vi "AutoEject.vi"(8 "error in (no error)":errorcluster, 9 "Time":dbl, 10 "Left Flywheel DevRef":T1={"DeviceStatus"={"status"=FALSE, "code"=0, "source"=""}, "Type"=enum."PWM", "PWM"={"PWM Channel"=enum."Invalid", "DeadBand"={"Name"="", "maxPositivePwm"=0, "minPositivePwm"=0, "centerPwm"=0, "maxNegativePwm"=0, "minNegativePwm"=0, "angularRange"=0}}, "CAN"={"Device Number"=0, "SetOutput VI Ref"=variant, "GetOutput VI Ref"=variant, "Enable VI Ref"=variant, "Disable VI Ref"=variant, "Data"=variant}, "Invert"=FALSE, "DIO PWM"={"PWM \"Enable\" Channel"=enum."Invalid", "DIOChannel"=enum."Invalid", "PWM Rate"=0.0}}, 11 "Right Flywheel DevRef":T1={"DeviceStatus"={"status"=FALSE, "code"=0, "source"=""}, "Type"=enum."PWM", "PWM"={"PWM Channel"=enum."Invalid", "DeadBand"={"Name"="", "maxPositivePwm"=0, "minPositivePwm"=0, "centerPwm"=0, "maxNegativePwm"=0, "minNegativePwm"=0, "angularRange"=0}}, "CAN"={"Device Number"=0, "SetOutput VI Ref"=variant, "GetOutput VI Ref"=variant, "Enable VI Ref"=variant, "Disable VI Ref"=variant, "Data"=variant}, "Invert"=FALSE, "DIO PWM"={"PWM \"Enable\" Channel"=enum."Invalid", "DIOChannel"=enum."Invalid", "PWM Rate"=0.0}}) -> (0 "error out":errorcluster)   [LabVIEW 2017]
uses:
  <vilib>/Rock Robotics/WPI/MotorControl/WPI_MotorControlDeviceRef.ctl
  <vilib>/Rock Robotics/WPI/MotorControl/WPI_MotorControlType.ctl
  <vilib>/Rock Robotics/SystemInterfaces/DIO/FPGA_DIOPWMChannel.ctl
  <vilib>/Rock Robotics/WPI/PWM/WPI_PWMDeadband.ctl
  <vilib>/Rock Robotics/SystemInterfaces/DIO/FPGA_DIOChannel.ctl
  <vilib>/Rock Robotics/WPI/ThirdParty/Phoenix-LabVIEW/Motor Controller/Controls/CTRE_Phoenix_MotorControl_ControlMode.ctl
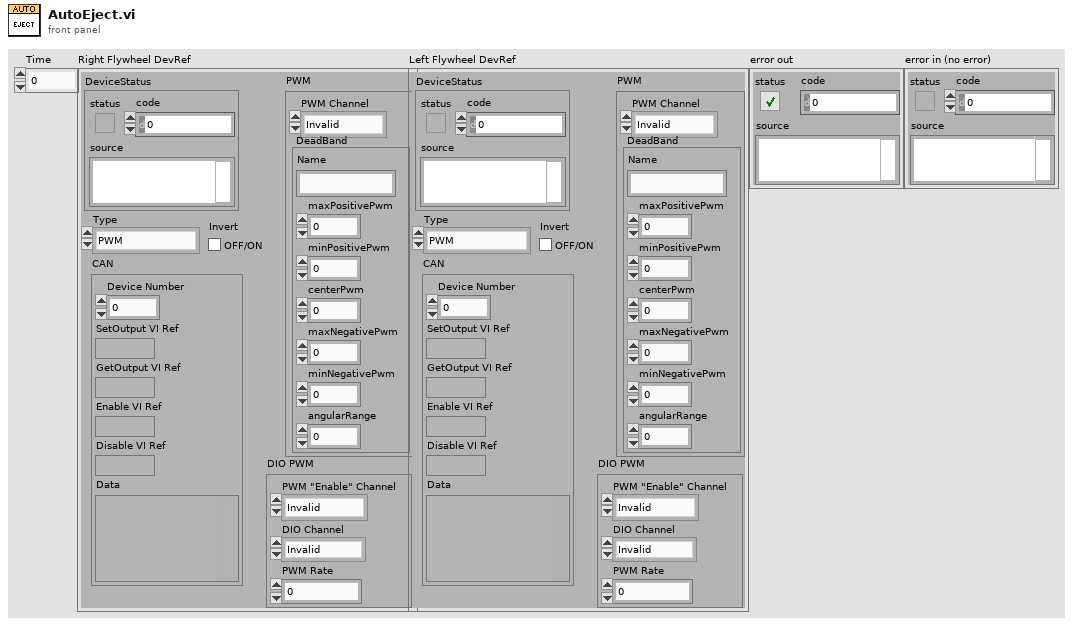
[diagram p1: front panel]
types:
  T1 = typedef "WPI_MotorControlDeviceRef.ctl" = cluster{"DeviceStatus":errorcluster, "Type":T2, "PWM":cluster{"PWM Channel":T3, "DeadBand":T4}, "CAN":cluster{"Device Number":u8, "SetOutput VI Ref":variant, "GetOutput VI Ref":variant, "Enable VI Ref":variant, "Disable VI Ref":variant, "Data":variant}, "Invert":bool, "DIO PWM":cluster{"PWM \"Enable\" Channel":T3, "DIOChannel":T5, "PWM Rate":dbl}}
  T2 = typedef "WPI_MotorControlType.ctl" = enum16{"PWM", "CAN", "DIO PWM"}
  T3 = typedef "FPGA_DIOPWMChannel.ctl" = enum8{"PWM 0", "PWM 1", "PWM 2", "PWM 3", "PWM 4", "PWM 5", "PWM 6", "PWM 7", "PWM 8", "PWM 9", "PWM MXP 0", "PWM MXP 1", "PWM MXP 2", "PWM MXP 3", "PWM MXP 4", "PWM MXP 5", "PWM MXP 6", "PWM MXP 7", "PWM MXP 8", "PWM MXP 9", "Invalid"}
  T4 = typedef "WPI_PWMDeadband.ctl" = cluster{"Name":string, "maxPositivePwm":i32, "minPositivePwm":i32, "centerPwm":i32, "maxNegativePwm":i32, "minNegativePwm":i32, "angularRange":u16}
  T5 = typedef "FPGA_DIOChannel.ctl" = enum8{"DIO 0", "DIO 1", "DIO 2", "DIO 3", "DIO 4", "DIO 5", "DIO 6", "DIO 7", "DIO 8", "DIO 9", "DIO MXP 0", "DIO MXP 1", "DIO MXP 2", "DIO MXP 3", "DIO MXP 4", "DIO MXP 5", "DIO MXP 6", "DIO MXP 7", "DIO MXP 8", "DIO MXP 9", "DIO MXP 10", "DIO MXP 11", "DIO MXP 12", "DIO MXP 13", "DIO MXP 14", "DIO MXP 15", "SPI Port CS1", "SPI Port CS2", "SPI Port CS3", "SPI Port MISO", "SPI Port MOSI", "Invalid"}
  T6 = typedef "CTRE_Phoenix_MotorControl_ControlMode.ctl" = u16
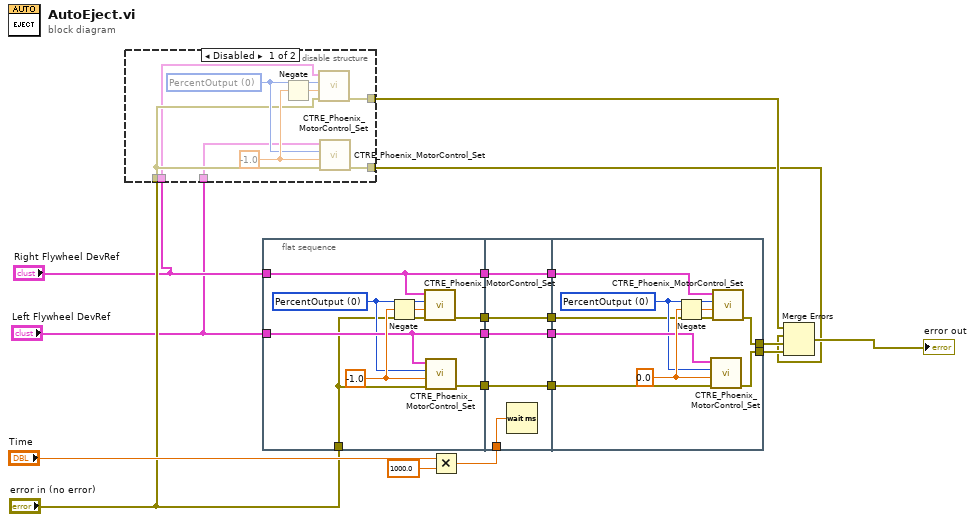
[diagram p0: block diagram]
diagram:
  n1 = disable-structure shown="Disabled" {
    disable-tunnel: "error in (no error)" -> [w24 _]
    disable-tunnel: "Right Flywheel DevRef" -> [w23 _]
    disable-tunnel: "Left Flywheel DevRef" -> [w22 _]
    disable-tunnel: [w21 _] -> w12
    disable-tunnel: [w20 _] -> w11
    frame Disabled {
      w25 = T6 0 items=["PercentOutput"=0, "Position"=1, "Velocity"=2, "Current"=3, "Follower"=5, "MotionProfile"=6, "MotionMagic"=7, "MotionMagicArc"=8, "MotionProfileArc"=10, "Disabled"=15] ("Control Mode")
      w27 = -1.0 ("Output")
      n2 = Negate(x=w27) -> (-x=w26:dbl)
      n3 = call <vilib>:"CTRE_Phoenix_MotorControl_Set.vi"("error in (no error)"=w24, "Output"=w26, "Control Mode"=w25, "PhoenixMotorControlDevRef"=w23) -> ("error out"=w21:errorcluster)  [unwired: 6 in, 1 out]
      n4 = call <vilib>:"CTRE_Phoenix_MotorControl_Set.vi"("error in (no error)"=w24, "Output"=w27, "Control Mode"=w25, "PhoenixMotorControlDevRef"=w22) -> ("error out"=w20:errorcluster)  [unwired: 6 in, 1 out]
    }
    frame Enabled {
    }
  }
  n5 = flat-sequence {
    tunnel: "Right Flywheel DevRef" -> [w33]
    tunnel: "Left Flywheel DevRef" -> [w32]
    tunnel: [w33] -> w10
    tunnel: [w32] -> w9
    tunnel: [w30] -> w8
    tunnel: [w29] -> w7
    tunnel: "error in (no error)" -> [w28]
    tunnel: [w40] -> w6
    tunnel: w10 -> [w40]
    tunnel: [w39] -> w5
    tunnel: w9 -> [w39]
    tunnel: w1 -> [w38]
    tunnel: [w37] -> w4
    tunnel: w8 -> [w37]
    tunnel: [w36] -> w3
    tunnel: w7 -> [w36]
    tunnel: w6 -> [w47]
    tunnel: w5 -> [w46]
    tunnel: w4 -> [w44]
    tunnel: w3 -> [w43]
    tunnel: [w42] -> w18
    tunnel: [w41] -> w17
    frame #0 {
      w31 = T6 0 items=["PercentOutput"=0, "Position"=1, "Velocity"=2, "Current"=3, "Follower"=5, "MotionProfile"=6, "MotionMagic"=7, "MotionMagicArc"=8, "MotionProfileArc"=10, "Disabled"=15] ("Control Mode")
      w35 = -1.0 ("Output")
      n6 = Negate(x=w35) -> (-x=w34:dbl)
      n7 = call <vilib>:"CTRE_Phoenix_MotorControl_Set.vi"("error in (no error)"=w28, "Output"=w34, "Control Mode"=w31, "PhoenixMotorControlDevRef"=w33) -> ("error out"=w29:errorcluster)  [unwired: 6 in, 1 out]
      n8 = call <vilib>:"CTRE_Phoenix_MotorControl_Set.vi"("error in (no error)"=w28, "Output"=w35, "Control Mode"=w31, "PhoenixMotorControlDevRef"=w32) -> ("error out"=w30:errorcluster)  [unwired: 6 in, 1 out]
    }
    frame #1 {
      n9 = Wait (ms)(milliseconds to wait=w38) -> ()  [unwired: 1 out]
    }
    frame #2 {
      w45 = T6 0 items=["PercentOutput"=0, "Position"=1, "Velocity"=2, "Current"=3, "Follower"=5, "MotionProfile"=6, "MotionMagic"=7, "MotionMagicArc"=8, "MotionProfileArc"=10, "Disabled"=15] ("Control Mode")
      w49 = 0.0 ("Output")
      n10 = Negate(x=w49) -> (-x=w48:dbl)
      n11 = call <vilib>:"CTRE_Phoenix_MotorControl_Set.vi"("error in (no error)"=w44, "Output"=w49, "Control Mode"=w45, "PhoenixMotorControlDevRef"=w46) -> ("error out"=w41:errorcluster)  [unwired: 6 in, 1 out]
      n12 = call <vilib>:"CTRE_Phoenix_MotorControl_Set.vi"("error in (no error)"=w43, "Output"=w48, "Control Mode"=w45, "PhoenixMotorControlDevRef"=w47) -> ("error out"=w42:errorcluster)  [unwired: 6 in, 1 out]
    }
  }
  n13 = Multiply(x="Time", y=1000.0) -> (x*y=w1:dbl)
  n14 = Merge Errors(w12, w11, w18, w17) -> (→"error out":errorcluster)
